vi "NML Bus Scan Metrolab Digital Integrator.vi"(3 "error in (no error)":errorcluster, 4 "String Read In":string, 5 "VISA Session":refnum<visa-resource-name>) -> (0 "error out":errorcluster, 1 "String Read Out":string, 2 "VISA Session Out":refnum<visa-resource-name>)   [LabVIEW 2024]
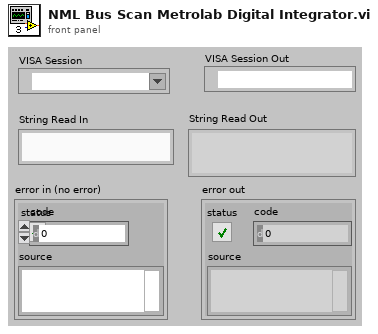
[diagram p1: front panel]
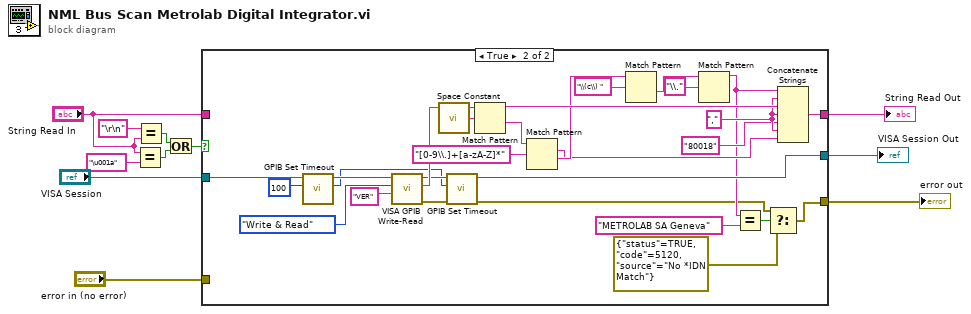
[diagram p0: block diagram]
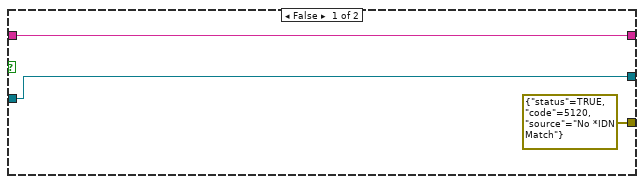
[diagram p2: hidden frame]
diagram:
  n1 = Equal?(x="String Read In", y="\u001a") -> (x = y?=w5:bool)
  n2 = Equal?(x="\r\n" ("y"), y="String Read In") -> (x = y?=w1:bool)
  n3 = Or(x=w1, y=w5) -> (x .or. y?=w2:bool)
  n4 = case shown="True" w2 {
    tunnel: [errorcluster {"status"=TRUE, "code"=5120, "source"="No *IDN Match"} ("error out") w16] -> w11
    tunnel: [w14 w27] -> w10
    tunnel: [w13 w21] -> w9
    tunnel: "VISA Session" -> [w13 w38]
    tunnel: "String Read In" -> [w14 _]
    tunnel: "error in (no error)" -> [_ _]
    frame False {
    }
    frame True {
      w23 = "," ("format string")
      n5 = call "GPIB Set Timeout.vi"("Timeout"=u32 100 ("General Settings:Timeout Value"), "VISA resource name"=w38) -> ("Old Timeout"=w34:u32, "dup VISA resource name"=w37:refnum<visa-resource-name>)  [unwired: 3 in, 1 out]
      n6 = call "VISA GPIB Write-Read.vi"("Command"="VER" ("String to Write"), "Action"=enum16{"Write", "Read", "Write & Read"}."Write & Read", "VISA resource name"=w37) -> ("error out"=w33:errorcluster, "String Returned"=w39:string, "dup VISA Session"=w36:refnum<visa-resource-name>)  [unwired: 5 in, 1 out]
      n7 = call <vilib>:"Space Constant.vi"() -> ("String"=w40:string)
      n8 = call "GPIB Set Timeout.vi"("Error In"=w33, "Timeout"=w34, "VISA resource name"=w36) -> ("Error Out"=w17:errorcluster, "dup VISA resource name"=w21:refnum<visa-resource-name>)  [unwired: 2 in, 1 out]
      n9 = Match Pattern(string=w39, regular expression=w40) -> (before substring=w31:string, after substring=w32:string)  [unwired: 1 in, 2 out]
      n10 = Match Pattern(string=w32, regular expression="[0-9\\.]+[a-zA-Z]*") -> (match substring=w24:string, after substring=w29:string)  [unwired: 1 in, 2 out]
      n11 = Match Pattern(string=w29, regular expression="\\(c\\) ") -> (after substring=w26:string)  [unwired: 1 in, 3 out]
      n12 = Match Pattern(string=w26, regular expression="\\.") -> (before substring=w20:string)  [unwired: 1 in, 3 out]
      n13 = Equal?(x=w20, y="METROLAB SA Geneva") -> (x = y?=w18:bool)
      n14 = Select(t=w17, s=w18, f=errorcluster {"status"=TRUE, "code"=5120, "source"="No *IDN Match"}) -> (s? t:f=w16:errorcluster)
      n15 = Concatenate Strings(w20, w23, w31, w23, "80018" ("string"), w23, w24) -> (w27:string)
    }
  }
  "error out" <- w11
  "String Read Out" <- w10
  "VISA Session Out" <- w9
